vi "Tetris New.vi"() -> ()   [LabVIEW 2019]
panel:
  out "wait mS":u16=250
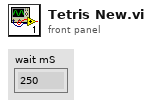
[diagram p1: front panel]
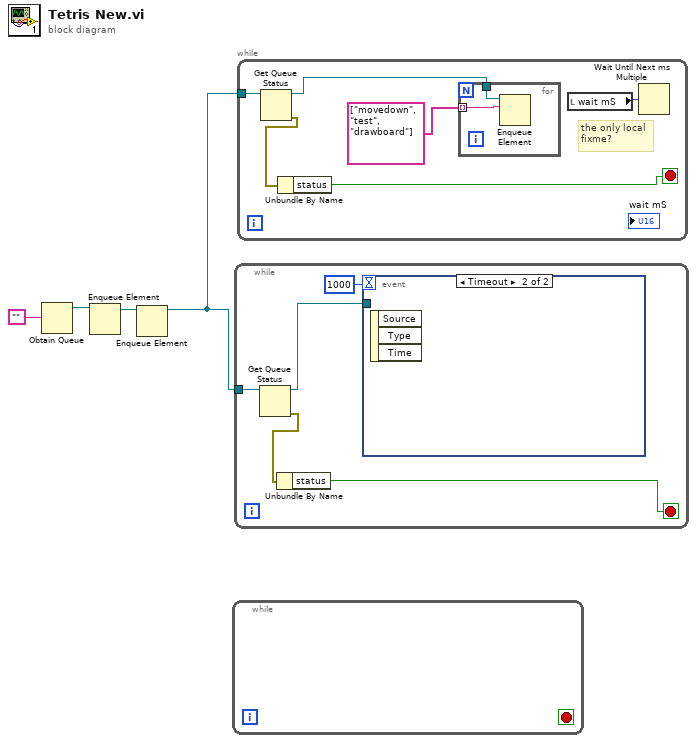
[diagram p0: block diagram]
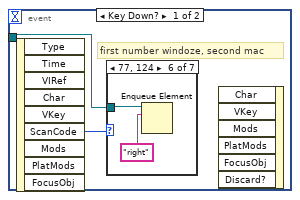
[diagram p2: hidden frame]
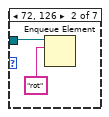
[diagram p4: hidden frame]
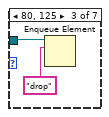
[diagram p5: hidden frame]
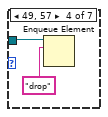
[diagram p6: hidden frame]
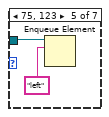
[diagram p7: hidden frame]
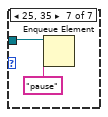
[diagram p8: hidden frame]
diagram:
  n1 = Obtain Queue(element data type="") -> (queue out=w2:refnum<queue>)  [unwired: 4 in, 2 out]
  n2 = Enqueue Element(queue=w2) -> (queue out=w3:refnum<queue>)  [unwired: 3 in, 2 out]
  n3 = Enqueue Element(queue=w3) -> (queue out=w1:refnum<queue>)  [unwired: 3 in, 2 out]
  n4 = while {
    stop <- _ stop-if-true
  }
  n5 = while {
    tunnel: w1 -> [w9]
    stop <- w6 stop-if-true
    n6 = Get Queue Status(queue=w9) -> (queue out=w8:refnum<queue>, error out=w7:errorcluster)  [unwired: 2 in, 6 out]
    n7 = Unbundle By Name(w7) -> ("status"=w6:bool)
    n8 = event shown="[1] Timeout" {
      selector: _ -> [_ _]
      dyn-events: _ -> [_ _]
      timeout: 1000 -> [_ _]
      tunnel: w8 -> [w10 _]
      event Key Down? {
        # "first number windoze, second mac"
        n9 = event-data() -> ("ScanCode"=w11:i16)  [unwired: 1 in, 8 out]
        n10 = case shown="77, 124" w11 {
          tunnel: w10 -> [_ w13 w15 w17 w19 w21 w23]
          frame 0, Default {
          }
          frame 72, 126 {
            n11 = Enqueue Element(queue=w13, element="rot") -> ()  [unwired: 2 in, 3 out]
          }
          frame 80, 125 {
            n12 = Enqueue Element(queue=w15, element="drop") -> ()  [unwired: 2 in, 3 out]
          }
          frame 49, 57 {
            n13 = Enqueue Element(queue=w17, element="drop") -> ()  [unwired: 2 in, 3 out]
          }
          frame 75, 123 {
            n14 = Enqueue Element(queue=w19, element="left") -> ()  [unwired: 2 in, 3 out]
          }
          frame 77, 124 {
            n15 = Enqueue Element(queue=w21, element="right") -> ()  [unwired: 2 in, 3 out]
          }
          frame 25, 35 {
            n16 = Enqueue Element(queue=w23, element="pause") -> ()  [unwired: 2 in, 3 out]
          }
        }
        n17 = event-data() -> ()  [unwired: 7 in, 1 out]
      }
      event Timeout {
        n18 = event-data() -> ()  [unwired: 1 in, 3 out]
      }
    }
  }
  n19 = while {
    tunnel: w1 -> [w25]
    stop <- w29 stop-if-true
    # "the only local\nfixme?"
    n20 = Get Queue Status(queue=w25) -> (queue out=w26:refnum<queue>, error out=w24:errorcluster)  [unwired: 2 in, 6 out]
    n21 = Unbundle By Name(w24) -> ("status"=w29:bool)
    n22 = for {
      tunnel: string[] ["movedown", "test", "drawboard"] -> [w31] mode=indexing
      tunnel: w26 -> [w30]
      n23 = Enqueue Element(queue=w30, element=w31) -> ()  [unwired: 2 in, 3 out]
    }
    n24 = local read "wait mS"() -> (w28:u16)
    n25 = Wait Until Next ms Multiple(millisecond multiple=w28) -> ()  [unwired: 1 out]
  }
